vi "Read J1939 Network Address.vi"(8 "error in (no error)":errorcluster, 11 "database file in":refnum<class "database file.lvclass">) -> (0 "error out":errorcluster, 2 "J1939 Network Address":u8, 3 "database file out":refnum<class "database file.lvclass">)   [LabVIEW 2013, in "database file.lvclass"]
uses:
  database file.lvclass
  database file.lvclass/database file.ctl
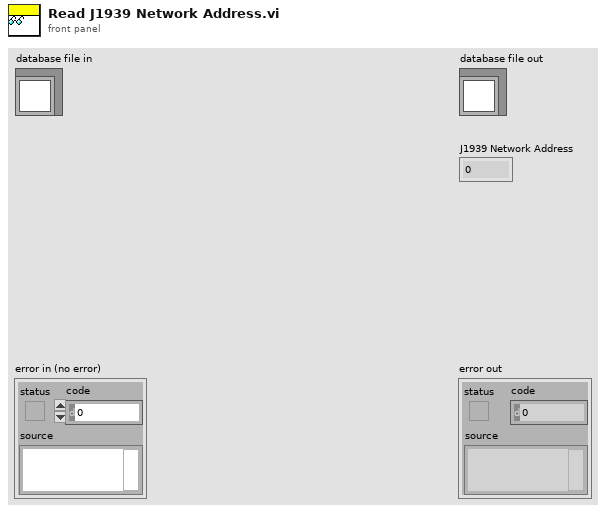
[diagram p1: front panel]
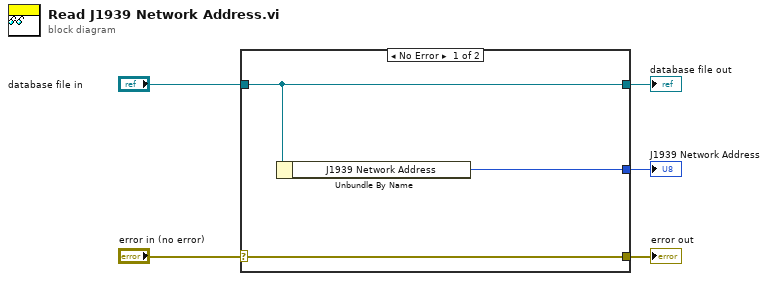
[diagram p0: block diagram]
diagram:
  n1 = case shown="No Error" "error in (no error)" {
    selector: "error in (no error)" -> [w8 w9]
    tunnel: [w8 w9] -> w4
    tunnel: [w7 w10] -> w2
    tunnel: "database file in" -> [w7 w10]
    tunnel: [w6 _] -> w1
    frame No Error {
      n2 = Unbundle By Name(w7) -> ("J1939 Network Address"=w6:u8)
    }
    frame Error {
    }
  }
  "error out" <- w4
  "database file out" <- w2
  "J1939 Network Address" <- w1
